vi "dfd_Elliptic Functions.vi"(0 "u":dbl=1.0 format="%.2f", 1 "k'":dbl=1.0 format="%.2f") -> (2 "convergence":bool=TRUE, 3 "sn(k)":dbl format="%.4f", 4 "cn(k)":dbl format="%.4f", 5 "dn(k)":dbl format="%.4f")   [LabVIEW 2017, in "NI_DigFilter_Design.lvlib"]
uses:
  <vilib>/addons/Digital Filter Design/NI_DigFilter_Design.lvlib
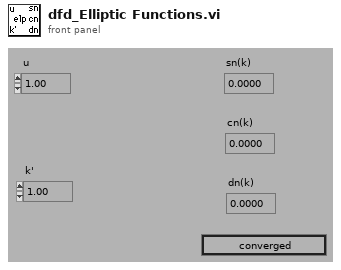
[diagram p1: front panel]
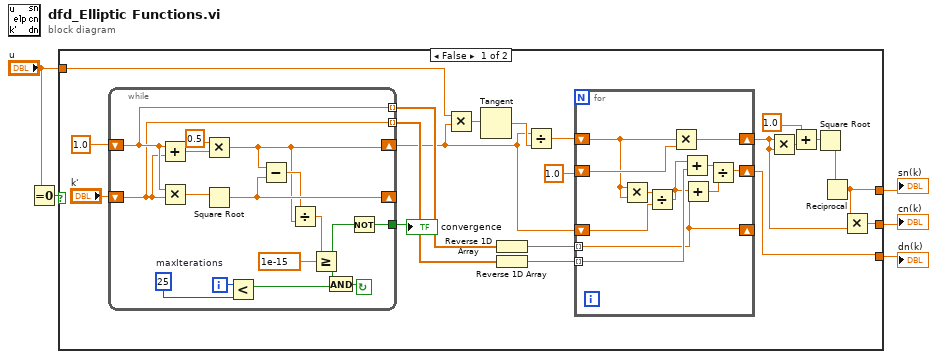
[diagram p0: block diagram]
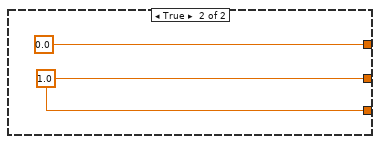
[diagram p2: hidden frame]
diagram:
  n1 = Equal To 0?(x="u") -> (x = 0?=w4:bool)
  n2 = case shown="False" w4 {
    tunnel: "u" -> [w24 _]
    tunnel: [w7 w55] -> w3
    tunnel: [w8 w55] -> w2
    tunnel: [w6 0.0] -> w1
    frame False {
      n3 = while {
        tunnel: [w28] -> w17 mode=indexing
        tunnel: [w29] -> w18 mode=indexing
        tunnel: [w31] -> w23
        shift-left: "k'" -> [w28]
        shift-right: [w39] -> _
        shift-left: 1.0 -> [w29]
        shift-right: [w37] -> w14
        i -> [w27]
        stop <- w32 continue-if-true
        w30 = 25  # maxIterations
        n4 = Add(x=w29, y=w28) -> (x+y=w41:dbl)
        n5 = Multiply(x=w29, y=w28) -> (x*y=w40:dbl)
        n6 = Multiply(x=0.5, y=w41) -> (x*y=w37:dbl)
        n7 = Square Root(x=w40) -> (sqrt(x)=w39:dbl)
        n8 = Less?(x=w27, y=w30) -> (x < y?=w33:bool)
        n9 = Subtract(x=w37, y=w39) -> (x-y=w38:dbl)
        n10 = Divide(x=w38, y=w37) -> (x/y=w35:dbl)
        n11 = Greater Or Equal?(x=w35, y=1e-15) -> (x >= y?=w34:bool)
        n12 = And(x=w34, y=w33) -> (x .and. y?=w32:bool)
        n13 = Not(x=w34) -> (.not. x?=w31:bool)
      }
      "convergence" <- w23
      n14 = Multiply(x=w24, y=w14) -> (x*y=w25:dbl)
      n15 = Tangent(1:w25) -> (0:w26:dbl)
      n16 = Reverse 1D Array(array=w18) -> (reversed array=w16:dbl[])
      n17 = Reverse 1D Array(array=w17) -> (reversed array=w15:dbl[])
      n18 = Divide(x=w14, y=w26) -> (x/y=w20:dbl)
      n19 = for {
        shift-right: [w52] -> w9
        shift-left: w20 -> [w51]
        shift-right: [w47] -> w7
        shift-left: 1.0 -> [w53]
        tunnel: w16 -> [w44] mode=indexing
        tunnel: w15 -> [w46] mode=indexing
        shift-right: [w44] -> _
        shift-left: w14 -> [w49]
        n20 = Multiply(x=w51, y=w51) -> (x*y=w50:dbl)
        n21 = Divide(x=w50, y=w49) -> (x/y=w45:dbl)
        n22 = Multiply(x=w51, y=w53) -> (x*y=w52:dbl)
        n23 = Add(x=w45, y=w46) -> (x+y=w48:dbl)
        n24 = Add(x=w45, y=w44) -> (x+y=w43:dbl)
        n25 = Divide(x=w48, y=w43) -> (x/y=w47:dbl)
      }
      n26 = Multiply(x=w9, y=w9) -> (x*y=w12:dbl)
      n27 = Add(x=1.0, y=w12) -> (x+y=w11:dbl)
      n28 = Square Root(x=w11) -> (sqrt(x)=w10:dbl)
      n29 = Reciprocal(x=w10) -> (1/x=w6:dbl)
      n30 = Multiply(x=w6, y=w9) -> (x*y=w8:dbl)
    }
    frame True {
      w55 = 1.0
    }
  }
  "sn(k)" <- w1
  "dn(k)" <- w3
  "cn(k)" <- w2
